vi "CSDB_Config.edit instances.vi"(1 "Classname":string, 2 "Names":string[](array[string]), 3 "Attributes":string[](array[string]), 4 "Values":string[][](array[string]), 5 "error in (no error)":errorcluster, 10 "new instances?":bool) -> (19 "error out":errorcluster)   [LabVIEW 2014, in "CSDB_Config.lvlib"]
doc: "This is a GUI that allows for editing attribute data of an object."
uses:
  CSDB_Config.lvlib
  CSDB_Common/CSDB_Common.lvlib
panel:
  out "type":string
  in  "set bool values":bool
  in  "set number  values":bool
  in  "set Shared Variable values":bool
  in  "apply mapping":bool
  in  "Cancel Button":bool
  in  "DONE":bool
  in  "set values":bool
  in  "Attribute":u16(ring) items=["Address0", "Address1", "Address10", "Address11", "Address12", "Address13", "Address14", "Address15", "Address2", "Address3", "Address4", "Address5", "Address5", "Address6", "Address7", "Address8", "Address9", "EventError", "EventTimeout", "Interface0", "Interface1", "Interface10", "Interface11", "Interface12", "Interface13", "Interface14", "Interface2", "Interface3", "Interface4", "Interface5", "Interface6", "Interface7", "Interface8", "Interface9", "PeriodicError", "PeriodicInterval", "PresetEvtWatchD", "PresetPdcWatchD", "Special0", "Special1", "Special10", "Special11", "Special12", "Special13", "Special14", "Special15", "Special2", "Special3", "Special4", "Special5", "Special6", "Special7", "Special8", "Special9", "SuperProc"]
  in  "Multicolumn Listbox":i32(listbox)
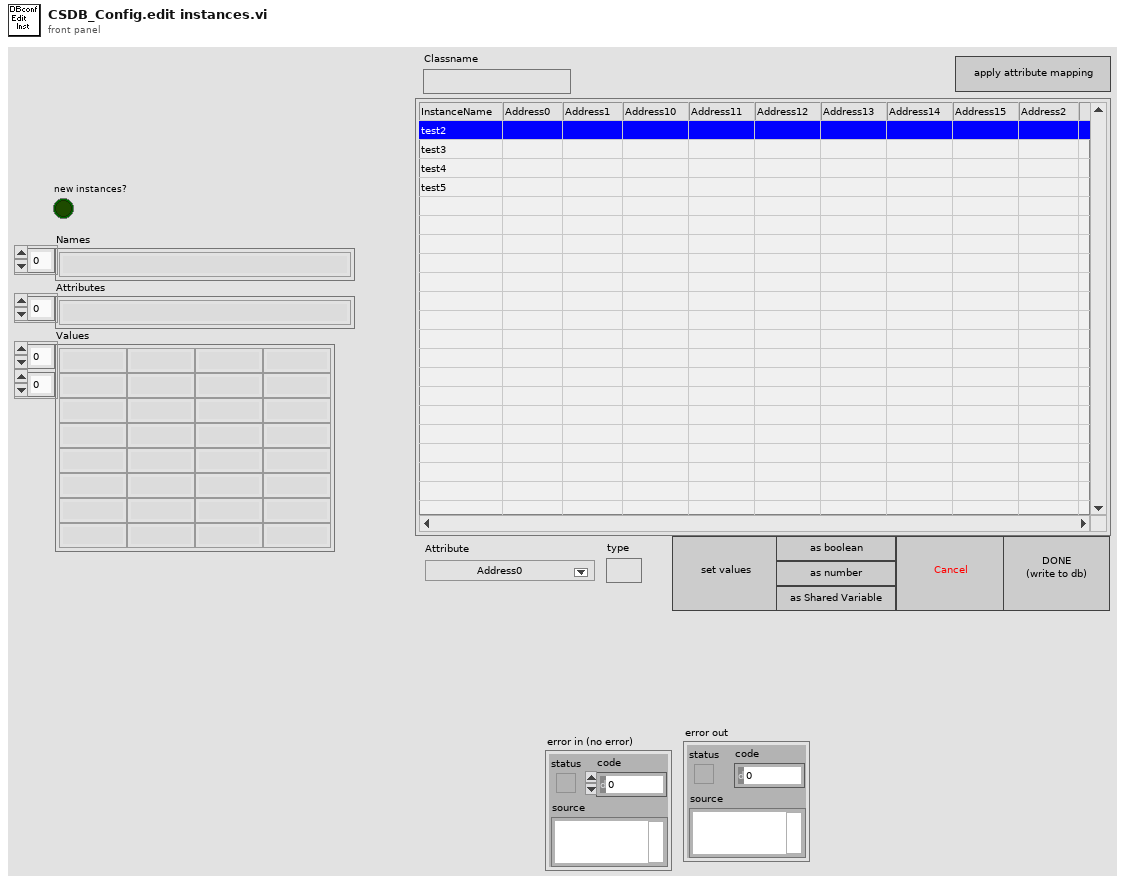
[diagram p1: front panel]
types:
  T1 = typedef "LVPoint32TypeDef.ctl" = cluster{"Horizontal":i32, "Vertical":i32}
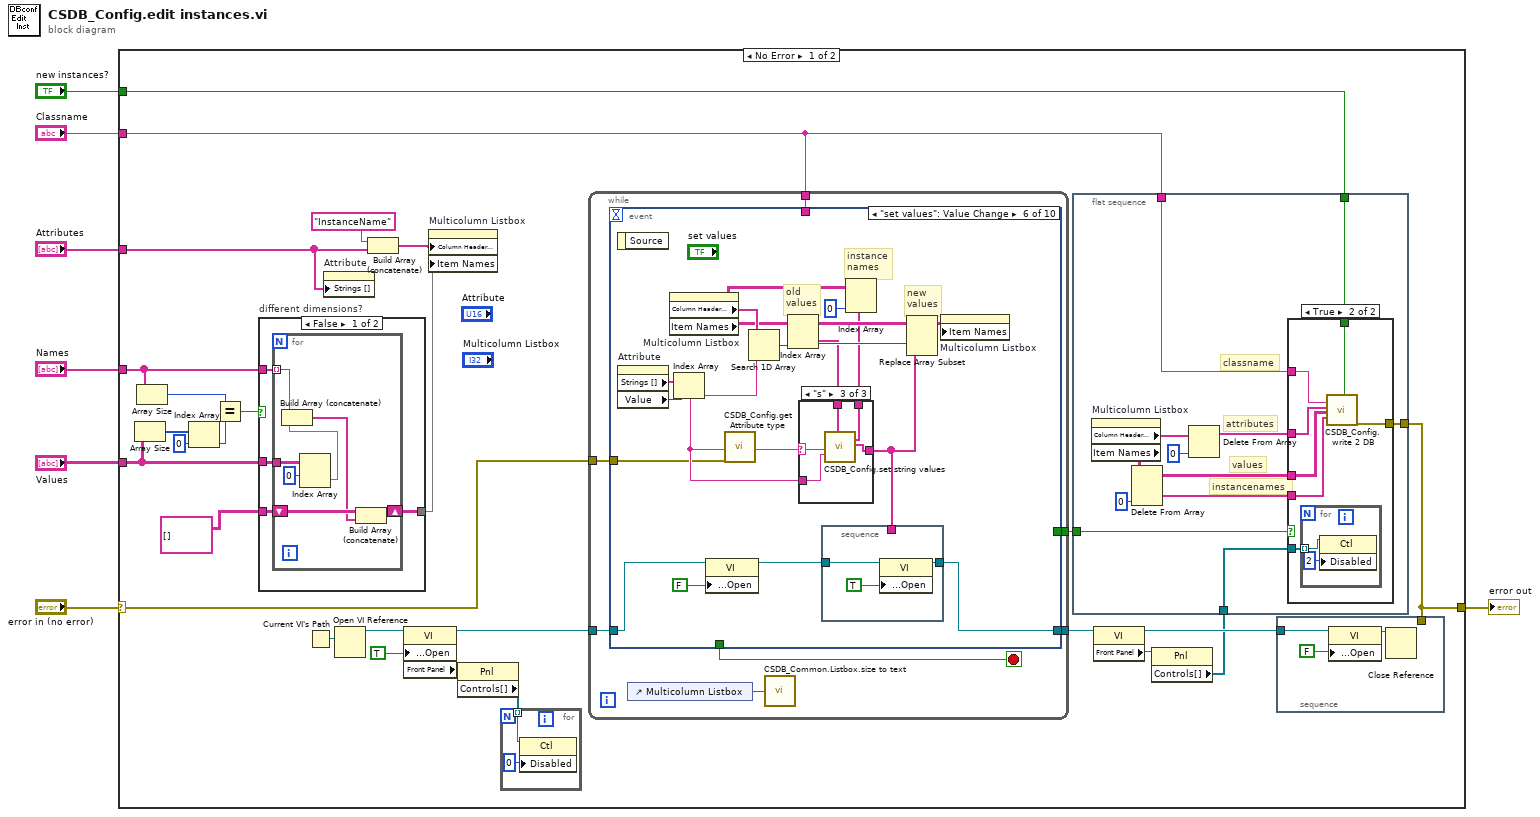
[diagram p0: block diagram]
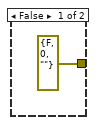
[diagram p2: hidden frame]
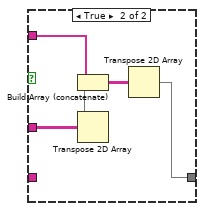
[diagram p3: hidden frame]
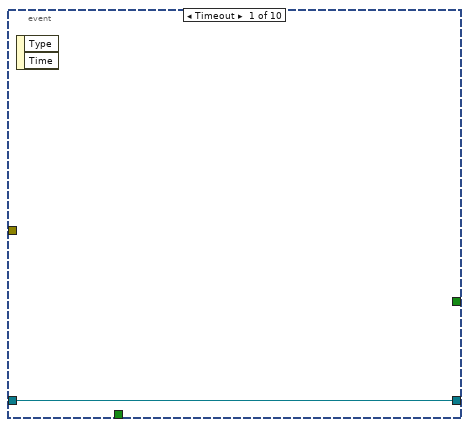
[diagram p4: hidden frame]
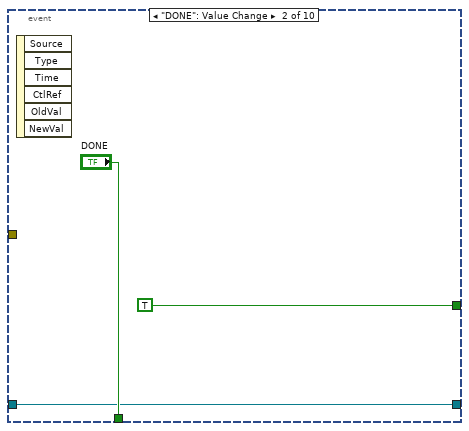
[diagram p5: hidden frame]
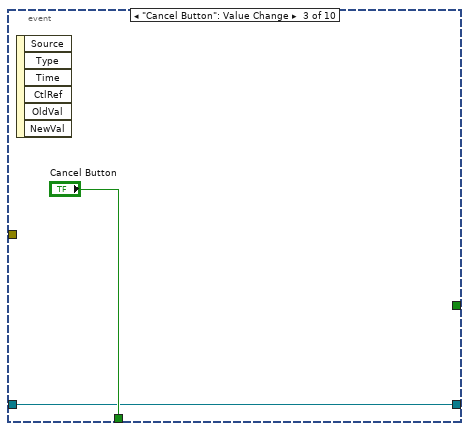
[diagram p6: hidden frame]
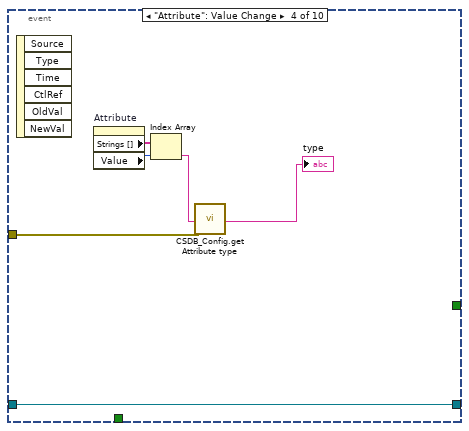
[diagram p7: hidden frame]
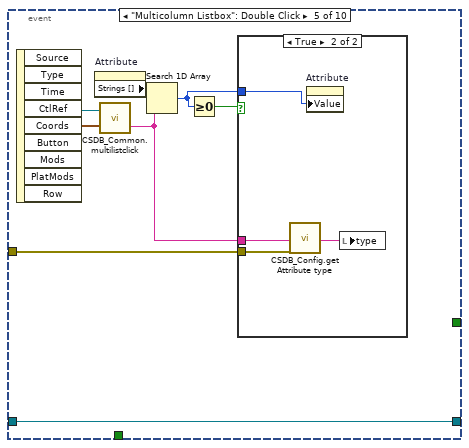
[diagram p8: hidden frame]
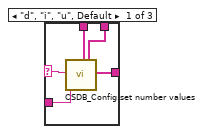
[diagram p10: hidden frame]
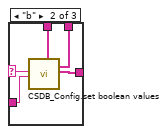
[diagram p11: hidden frame]
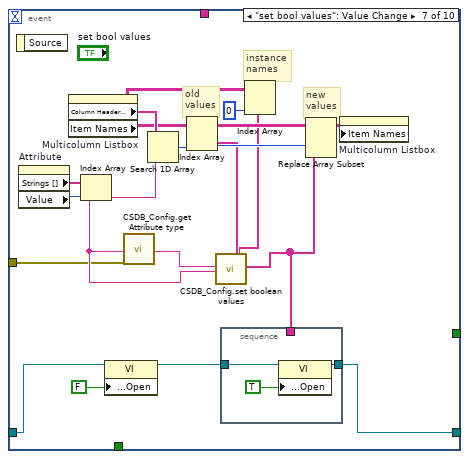
[diagram p12: hidden frame]
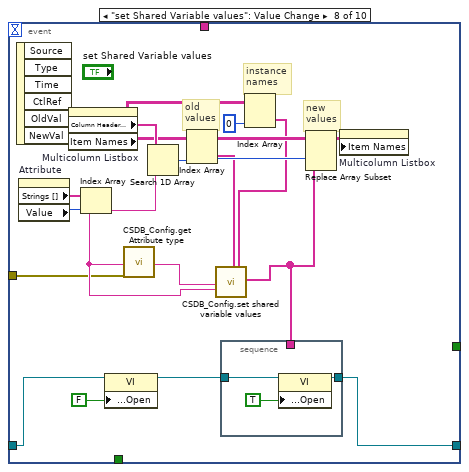
[diagram p13: hidden frame]
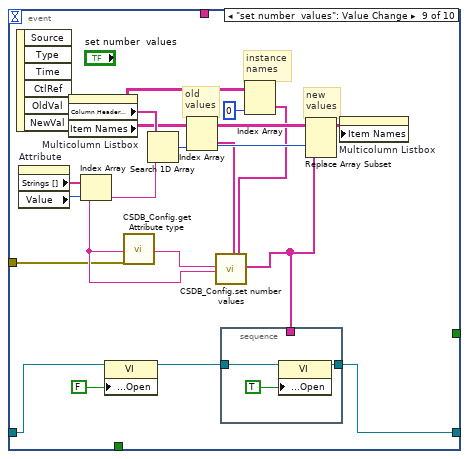
[diagram p14: hidden frame]
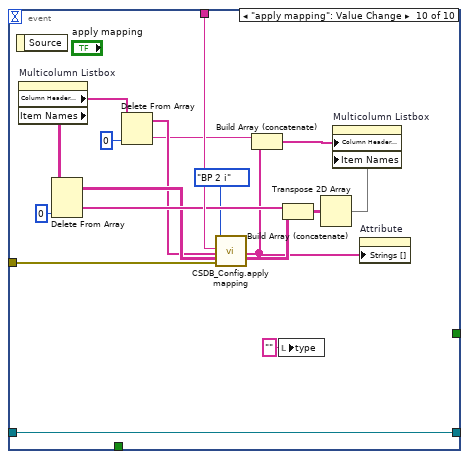
[diagram p15: hidden frame]
diagram:
  n1 = case shown="No Error" "error in (no error)" {
    selector: "error in (no error)" -> [w8 w222]
    tunnel: "Attributes" -> [w28 _]
    tunnel: "Names" -> [w22 _]
    tunnel: "Values" -> [w21 _]
    tunnel: [w18 w222] -> w4
    tunnel: "Classname" -> [w17 _]
    tunnel: "new instances?" -> [w15 _]
    frame No Error {
      n2 = Array Size(array=w21) -> (size(s)=w27:i32[])
      n3 = Array Size(array=w22) -> (size(s)=w25:i32)
      n4 = Index Array(array=w27, index=0) -> (element=w24:i32)
      n5 = Equal?(x=w25, y=w24) -> (x = y?=w23:bool)
      n6 = case "different dimensions?" shown="False" w23 {
        tunnel: w22 -> [w64 w77]
        tunnel: w21 -> [w65 w74]
        tunnel: [w62 w76] -> w20
        tunnel: string[][] [] -> [w63 _]
        frame False {
          n7 = for {
            tunnel: w65 -> [w72]
            tunnel: w64 -> [w71] mode=indexing
            shift-right: [w67] -> w62
            shift-left: w63 -> [w68]
            n8 = Index Array(array=w72, index (row)=0) -> (element=w69:string[])  [unwired: 1 in]
            n9 = Build Array (concatenate)(w71, w69) -> (w66:string[])
            n10 = Build Array (concatenate)(w68, w66) -> (w67:string[][])
          }
        }
        frame True {
          n11 = Transpose 2D Array(2D array=w74) -> (transposed array=w73:string[][])
          n12 = Build Array (concatenate)(w77, w73) -> (w75:string[][])
          n13 = Transpose 2D Array(2D array=w75) -> (transposed array=w76:string[][])
        }
      }
      n14 = Current VI's Path() -> (path=w32:path)
      n15 = property on="Attribute" class="Ring (strict)"("Strings []"=w28) -> ()  [unwired: 2 in, 2 out]
      n16 = Open VI Reference(vi path=w32) -> (vi reference=w31:refnum<vi>)  [unwired: 5 in, 1 out]
      n17 = Build Array (concatenate)("InstanceName", w28) -> (w33:string[])
      n18 = property class="VI"(reference=w31, "Front Panel Window:Open"=TRUE) -> (reference out=w29:refnum<vi>, "Front Panel"=w10:refnum<vi>)  [unwired: 1 in, 1 out]
      n19 = property on="Multicolumn Listbox" class="MCListbox (strict)"("Column Header Strings[]"=w33, "Item Names"=w20) -> ()  [unwired: 2 in, 2 out]
      n20 = property class="Pnl"(reference=w10) -> ("Controls[]"=w9:refnum<vi>[])  [unwired: 1 in, 2 out]
      n21 = for {
        tunnel: w9 -> [w35] mode=indexing
        n22 = property class="Ctl"(reference=w35, "Disabled"=u8 0) -> ()  [unwired: 1 in, 2 out]
      }
      n23 = while {
        tunnel: [w80] -> w13
        tunnel: w29 -> [w79]
        tunnel: w8 -> [w83]
        tunnel: [w82] -> w19
        tunnel: w17 -> [w81]
        stop <- w84 stop-if-true
        n24 = event shown="[5] \"set values\": Value Change" {
          selector: _ -> [_ _ _ _ _ _ _ _ _ _]
          dyn-events: _ -> [_ _ _ _ _ _ _ _ _ _]
          timeout: _ -> [_ _ _ _ _ _ _ _ _ _]
          tunnel: [_ "DONE" "Cancel Button" _ _ _ _ _ _ _] -> w84
          tunnel: w83 -> [_ _ _ w96 w102 w115 w151 w173 w193 w221]
          tunnel: [_ TRUE _ _ _ _ _ _ _ _] -> w82
          tunnel: w81 -> [_ _ _ _ _ _ _ _ _ w220]
          tunnel: [w85 w86 w89 w91 w97 w111 w147 w169 w189 w205] -> w80
          tunnel: w79 -> [w85 w86 w89 w91 w97 w113 w149 w171 w191 w205]
          event Timeout {
            n25 = event-data() -> ()  [unwired: 1 in, 2 out]
          }
          event "DONE": Value Change {
            n26 = event-data() -> ()  [unwired: 1 in, 6 out]
          }
          event "Cancel Button": Value Change {
            n27 = event-data() -> ()  [unwired: 1 in, 6 out]
          }
          event "Attribute": Value Change {
            n28 = event-data() -> ()  [unwired: 1 in, 6 out]
            n29 = property on="Attribute" class="Ring (strict)"() -> ("Strings []"=w94:string[], "Value"=w93:u16)  [unwired: 2 in, 2 out]
            n30 = Index Array(array=w94, index=w93) -> (element=w92:string)
            n31 = call "CSDB_Config.get Attribute type.vi"("AttributeName"=w92, "error in (no error)"=w96) -> ("Type"=→"type":string)  [unwired: 16 in, 1 out]
          }
          event "Multicolumn Listbox": Double Click {
            n32 = event-data() -> ("CtlRef"=w104:refnum<vi>, "Coords"=w103:T1)  [unwired: 1 in, 7 out]
            n33 = property on="Attribute" class="Ring (strict)"() -> ("Strings []"=w101:string[])  [unwired: 2 in, 2 out]
            n34 = call "CSDB_Common.multilistclick.vi"("Coords"=w103, "Multicolumn ref"=w104) -> ("header"=w100:string)  [unwired: 1 out]
            n35 = Search 1D Array(1D array=w101, element=w100) -> (index of element=w98:i32)  [unwired: 1 in]
            n36 = Greater Or Equal To 0?(x=w98) -> (x >= 0?=w99:bool)
            n37 = case shown="True" w99 {
              tunnel: w102 -> [_ w108]
              tunnel: w100 -> [_ w106]
              tunnel: w98 -> [_ w105]
              frame False {
              }
              frame True {
                n38 = call "CSDB_Config.get Attribute type.vi"("AttributeName"=w106, "error in (no error)"=w108) -> ("Type"=w107:string)  [unwired: 16 in, 1 out]
                n39 = property on="Attribute" class="Ring (strict)"("Value"=w105) -> ()  [unwired: 2 in, 2 out]
                n40 = local write "type"(w107) -> ()
              }
            }
          }
          event "set values": Value Change {
            # "new\nvalues"
            # "instance\nnames"
            # "old\nvalues"
            n41 = event-data() -> ()  [unwired: 1 in, 1 out]
            n42 = property on="Attribute" class="Ring (strict)"() -> ("Strings []"=w125:string[], "Value"=w109:u16)  [unwired: 2 in, 2 out]
            n43 = property on="Multicolumn Listbox" class="MCListbox (strict)"() -> ("Column Header Strings[]"=w123:string[], "Item Names"=w118:string[][])  [unwired: 2 in, 2 out]
            n44 = Index Array(array=w125, index=w109) -> (element=w119:string)
            n45 = property class="VI"(reference=w113, "Front Panel Window:Open"=FALSE) -> (reference out=w112:refnum<vi>)  [unwired: 1 in, 1 out]
            n46 = call "CSDB_Config.get Attribute type.vi"("AttributeName"=w119, "error in (no error)"=w115) -> ("Type"=w124:string)  [unwired: 16 in, 1 out]
            n47 = Search 1D Array(1D array=w123, element=w119) -> (index of element=w121:i32)  [unwired: 1 in]
            n48 = Index Array(array=w118, index (col)=w121) -> (element=w120:string[])  [unwired: 1 in]
            n49 = Index Array(array=w118, index (col)=0 ("disabled index (col)")) -> (element=w116:string[])  [unwired: 1 in]
            n50 = case shown="\"s\"" w124 {
              selector: w124 -> [w133 w135 w143]
              tunnel: [w130 w138 w142] -> w110
              tunnel: w120 -> [w131 w137 w141]
              tunnel: w119 -> [w132 w134 w139]
              tunnel: w116 -> [w129 w136 w140]
              frame "d", "i", "u", Default {
                n51 = call "CSDB_Config.set number values.vi"("Type"=w133, "Attribute"=w132, "Values in"=w131, "InstanceNames"=w129) -> ("Values out"=w130:string[])  [unwired: 15 in]
              }
              frame "b" {
                n52 = call "CSDB_Config.set boolean values.vi"("Type"=w135, "AttributeName"=w134, "Values in"=w137, "InstanceNames in"=w136) -> ("Values out"=w138:string[])  [unwired: 15 in]
              }
              frame "s" {
                n53 = call "CSDB_Config.set string values.vi"("Type"=w143, "AttributeName"=w139, "Values in"=w141, "InstanceNames in"=w140) -> ("Values out"=w142:string[])  [unwired: 15 in]
              }
            }
            n54 = stacked-sequence {
              tunnel: w112 -> [w127]
              tunnel: [w126] -> w111
              tunnel: w110 -> [_]
              frame #0 {
                n55 = property class="VI"(reference=w127, "Front Panel Window:Open"=TRUE) -> (reference out=w126:refnum<vi>)  [unwired: 1 in, 1 out]
              }
            }
            n56 = Replace Array Subset(array=w118, new element=w110, index (col)=w121) -> (w122:string[][])  [unwired: 1 in]
            n57 = property on="Multicolumn Listbox" class="MCListbox (strict)"("Item Names"=w122) -> ()  [unwired: 2 in, 2 out]
          }
          event "set bool values": Value Change {
            # "new\nvalues"
            # "instance\nnames"
            # "old\nvalues"
            n58 = event-data() -> ()  [unwired: 1 in, 1 out]
            n59 = property on="Attribute" class="Ring (strict)"() -> ("Strings []"=w145:string[], "Value"=w144:u16)  [unwired: 2 in, 2 out]
            n60 = property on="Multicolumn Listbox" class="MCListbox (strict)"() -> ("Column Header Strings[]"=w159:string[], "Item Names"=w154:string[][])  [unwired: 2 in, 2 out]
            n61 = Index Array(array=w145, index=w144) -> (element=w155:string)
            n62 = property class="VI"(reference=w149, "Front Panel Window:Open"=FALSE) -> (reference out=w148:refnum<vi>)  [unwired: 1 in, 1 out]
            n63 = call "CSDB_Config.get Attribute type.vi"("AttributeName"=w155, "error in (no error)"=w151) -> ("Type"=w160:string)  [unwired: 16 in, 1 out]
            n64 = Search 1D Array(1D array=w159, element=w155) -> (index of element=w157:i32)  [unwired: 1 in]
            n65 = Index Array(array=w154, index (col)=w157) -> (element=w156:string[])  [unwired: 1 in]
            n66 = Index Array(array=w154, index (col)=0 ("disabled index (col)")) -> (element=w152:string[])  [unwired: 1 in]
            n67 = call "CSDB_Config.set boolean values.vi"("Type"=w160, "AttributeName"=w155, "Values in"=w156, "InstanceNames in"=w152) -> ("Values out"=w146:string[])  [unwired: 15 in]
            n68 = stacked-sequence {
              tunnel: w148 -> [w162]
              tunnel: [w161] -> w147
              tunnel: w146 -> [_]
              frame #0 {
                n69 = property class="VI"(reference=w162, "Front Panel Window:Open"=TRUE) -> (reference out=w161:refnum<vi>)  [unwired: 1 in, 1 out]
              }
            }
            n70 = Replace Array Subset(array=w154, new element=w146, index (col)=w157) -> (w158:string[][])  [unwired: 1 in]
            n71 = property on="Multicolumn Listbox" class="MCListbox (strict)"("Item Names"=w158) -> ()  [unwired: 2 in, 2 out]
          }
          event "set Shared Variable values": Value Change {
            # "new\nvalues"
            # "instance\nnames"
            # "old\nvalues"
            n72 = event-data() -> ()  [unwired: 1 in, 6 out]
            n73 = property on="Attribute" class="Ring (strict)"() -> ("Strings []"=w167:string[], "Value"=w166:u16)  [unwired: 2 in, 2 out]
            n74 = property on="Multicolumn Listbox" class="MCListbox (strict)"() -> ("Column Header Strings[]"=w179:string[], "Item Names"=w175:string[][])  [unwired: 2 in, 2 out]
            n75 = Index Array(array=w167, index=w166) -> (element=w176:string)
            n76 = property class="VI"(reference=w171, "Front Panel Window:Open"=FALSE) -> (reference out=w170:refnum<vi>)  [unwired: 1 in, 1 out]
            n77 = call "CSDB_Config.get Attribute type.vi"("AttributeName"=w176, "error in (no error)"=w173) -> ("Type"=w180:string)  [unwired: 16 in, 1 out]
            n78 = Search 1D Array(1D array=w179, element=w176) -> (index of element=w177:i32)  [unwired: 1 in]
            n79 = Index Array(array=w175, index (col)=w177) -> (element=w165:string[])  [unwired: 1 in]
            n80 = Index Array(array=w175, index (col)=0 ("disabled index (col)")) -> (element=w164:string[])  [unwired: 1 in]
            n81 = call "CSDB_Config.set shared variable values.vi"("Type"=w180, "AttributeName"=w176, "Values in"=w165, "InstanceNames in"=w164) -> ("Values out"=w168:string[])  [unwired: 15 in]
            n82 = stacked-sequence {
              tunnel: w170 -> [w182]
              tunnel: [w181] -> w169
              tunnel: w168 -> [_]
              frame #0 {
                n83 = property class="VI"(reference=w182, "Front Panel Window:Open"=TRUE) -> (reference out=w181:refnum<vi>)  [unwired: 1 in, 1 out]
              }
            }
            n84 = Replace Array Subset(array=w175, new element=w168, index (col)=w177) -> (w178:string[][])  [unwired: 1 in]
            n85 = property on="Multicolumn Listbox" class="MCListbox (strict)"("Item Names"=w178) -> ()  [unwired: 2 in, 2 out]
          }
          event "set number  values": Value Change {
            # "new\nvalues"
            # "instance\nnames"
            # "old\nvalues"
            n86 = event-data() -> ()  [unwired: 1 in, 6 out]
            n87 = property on="Attribute" class="Ring (strict)"() -> ("Strings []"=w187:string[], "Value"=w186:u16)  [unwired: 2 in, 2 out]
            n88 = property on="Multicolumn Listbox" class="MCListbox (strict)"() -> ("Column Header Strings[]"=w199:string[], "Item Names"=w195:string[][])  [unwired: 2 in, 2 out]
            n89 = Index Array(array=w187, index=w186) -> (element=w196:string)
            n90 = property class="VI"(reference=w191, "Front Panel Window:Open"=FALSE) -> (reference out=w190:refnum<vi>)  [unwired: 1 in, 1 out]
            n91 = call "CSDB_Config.get Attribute type.vi"("AttributeName"=w196, "error in (no error)"=w193) -> ("Type"=w200:string)  [unwired: 16 in, 1 out]
            n92 = Search 1D Array(1D array=w199, element=w196) -> (index of element=w197:i32)  [unwired: 1 in]
            n93 = Index Array(array=w195, index (col)=w197) -> (element=w185:string[])  [unwired: 1 in]
            n94 = Index Array(array=w195, index (col)=0 ("disabled index (col)")) -> (element=w184:string[])  [unwired: 1 in]
            n95 = call "CSDB_Config.set number values.vi"("Type"=w200, "Attribute"=w196, "Values in"=w185, "InstanceNames"=w184) -> ("Values out"=w188:string[])  [unwired: 15 in]
            n96 = stacked-sequence {
              tunnel: w190 -> [w202]
              tunnel: [w201] -> w189
              tunnel: w188 -> [_]
              frame #0 {
                n97 = property class="VI"(reference=w202, "Front Panel Window:Open"=TRUE) -> (reference out=w201:refnum<vi>)  [unwired: 1 in, 1 out]
              }
            }
            n98 = Replace Array Subset(array=w195, new element=w188, index (col)=w197) -> (w198:string[][])  [unwired: 1 in]
            n99 = property on="Multicolumn Listbox" class="MCListbox (strict)"("Item Names"=w198) -> ()  [unwired: 2 in, 2 out]
          }
          event "apply mapping": Value Change {
            n100 = event-data() -> ()  [unwired: 1 in, 1 out]
            n101 = property on="Multicolumn Listbox" class="MCListbox (strict)"() -> ("Column Header Strings[]"=w212:string[], "Item Names"=w219:string[][])  [unwired: 2 in, 2 out]
            n102 = Delete From Array(array=w219, index (col)=0 ("disabled index (col)")) -> (deleted portion=w216:string[], array with subset deleted=w215:string[][])  [unwired: 2 in]
            n103 = Delete From Array(array=w212, index=0) -> (deleted portion=w209:string, array with subset deleted=w210:string[])  [unwired: 1 in]
            n104 = call "CSDB_Config.apply mapping.vi"("Enum"=enum16{"i 2 BP", "BP 2 i", "get"}."BP 2 i", "ClassName"=w220, "AttributeNamesIn"=w210, "Values in"=w215, "error in (no error)"=w221) -> ("AttributeNames out"=w208:string[], "Values out"=w217:string[][])  [unwired: 12 in, 1 out]
            n105 = Build Array (concatenate)(w209, w208) -> (w207:string[])
            n106 = local write "type"("" ("type")) -> ()
            n107 = Build Array (concatenate)(w216, w217) -> (w214:string[][])
            n108 = Transpose 2D Array(2D array=w214) -> (transposed array=w213:string[][])
            n109 = property on="Multicolumn Listbox" class="MCListbox (strict)"("Column Header Strings[]"=w207, "Item Names"=w213) -> ()  [unwired: 2 in, 2 out]
            n110 = property on="Attribute" class="Ring (strict)"("Strings []"=w208) -> ()  [unwired: 2 in, 2 out]
          }
        }
        n111 = control-ref of="Multicolumn Listbox"() -> (w78:refnum<vi>)
        n112 = call "CSDB_Common.Listbox.size to text.vi"("listbox ref"=w78) -> ()  [unwired: 2 in]
      }
      n113 = flat-sequence {
        tunnel: w19 -> [w41]
        tunnel: [w40] -> w18
        tunnel: w17 -> [w39]
        tunnel: w15 -> [w38]
        tunnel: w11 -> [w37]
        frame #0 {
          # "classname"
          # "instancenames"
          # "values"
          # "attributes"
          n114 = property on="Multicolumn Listbox" class="MCListbox (strict)"() -> ("Column Header Strings[]"=w46:string[], "Item Names"=w48:string[][])  [unwired: 2 in, 2 out]
          n115 = Delete From Array(array=w48, index (col)=0 ("disabled index (col)")) -> (deleted portion=w42:string[], array with subset deleted=w43:string[][])  [unwired: 2 in]
          n116 = Delete From Array(array=w46, index=0) -> (array with subset deleted=w44:string[])  [unwired: 1 in, 1 out]
          n117 = case shown="True" w41 {
            tunnel: w44 -> [_ w56]
            tunnel: w43 -> [_ w55]
            tunnel: w42 -> [_ w54]
            tunnel: w39 -> [_ w53]
            tunnel: [errorcluster {"status"=FALSE, "code"=0, "source"=""} ("error out") w52] -> w40
            tunnel: w38 -> [_ w51]
            tunnel: w37 -> [_ w50]
            frame False {
            }
            frame True {
              n118 = for {
                tunnel: w50 -> [w58] mode=indexing
                n119 = property class="Ctl"(reference=w58, "Disabled"=u8 2) -> ()  [unwired: 1 in, 2 out]
              }
              n120 = call "CSDB_Config.write 2 DB.vi"("ClassName"=w53, "AttributeNames"=w56, "Values"=w55, "InstanceNames"=w54, "new instances?"=w51) -> ("error out"=w52:errorcluster)  [unwired: 14 in]
            }
          }
        }
      }
      n121 = property class="VI"(reference=w13) -> (reference out=w14:refnum<vi>, "Front Panel"=w12:refnum<vi>)  [unwired: 1 in, 1 out]
      n122 = property class="Pnl"(reference=w12) -> ("Controls[]"=w11:refnum<vi>[])  [unwired: 1 in, 2 out]
      n123 = stacked-sequence {
        tunnel: w14 -> [w59]
        tunnel: w18 -> [_]
        frame #0 {
          n124 = property class="VI"(reference=w59, "Front Panel Window:Open"=FALSE) -> (reference out=w60:refnum<vi>)  [unwired: 1 in, 1 out]
          n125 = Close Reference(reference=w60) -> ()  [unwired: 1 in, 1 out]
        }
      }
    }
    frame Error {
    }
  }
  "error out" <- w4
